vi "test Call Mock Transceiver With Errors.vi"(8 "error in (no error)":errorcluster, 11 "TestCase in":refnum<class "Transceiver Test Cases.lvclass">) -> (0 "error out":errorcluster, 3 "TestCase out":refnum<class "Transceiver Test Cases.lvclass">)   [LabVIEW 2017, in "Transceiver Test Cases.lvclass"]
uses:
  Transceiver Test Cases.lvclass
  Configuration/Public/Controls/DSF Engine Transfer Group Configuration.ctl
  Configuration/Public/Controls/DSF Direction.ctl
  Configuration/Public/Controls/DSF Timing Info.ctl
  Configuration/Public/Controls/DSF Engine Transfer Configuration.ctl
  Configuration/Public/Controls/DSF Byte Order.ctl
  Configuration/Public/Controls/DSF Engine Channel Configuration.ctl
  Configuration/Public/Controls/DSF Data Type.ctl
  Configuration/Public/Controls/DSF Settings Info.ctl
  DSF Core.lvlib
  <vilib>/addons/_JKI Toolkits/VI Tester/TestCase.llb/TestCase.lvclass
  C:/Program Files (x86)/National Instruments/LabVIEW 2017/vi.lib/addons/_JKI Toolkits/VI Tester/TestCase.llb/TestCase.lvclass
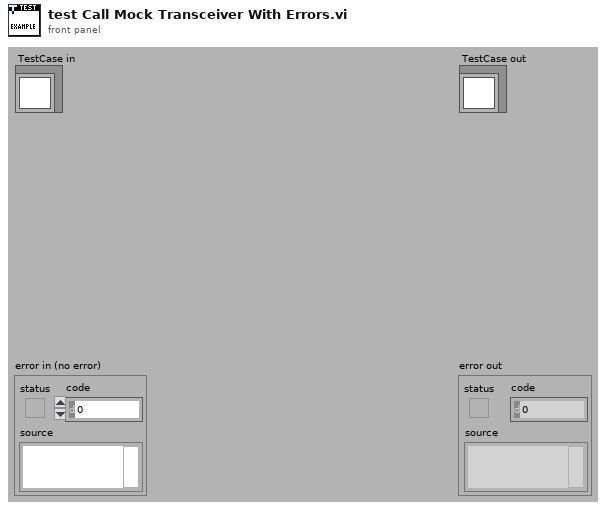
[diagram p1: front panel]
types:
  T1 = typedef "DSF Core.lvlib/DSF Engine Transfer Group Configuration.ctl" = cluster{"name":string, "direction":T2, "cycle timing":T3, "Transfers":T4[], "settings":T8}
  T2 = typedef "DSF Core.lvlib/DSF Direction.ctl" = enum8{"Tx", "Rx"}
  T3 = typedef "DSF Core.lvlib/DSF Timing Info.ctl" = cluster{"priority":u64, "decimation":u64, "offset":u64}
  T4 = typedef "DSF Core.lvlib/DSF Engine Transfer Configuration.ctl" = cluster{"name":string, "byte order":T5, "channel configurations":T6[], "settings":T8}
  T5 = typedef "DSF Core.lvlib/DSF Byte Order.ctl" = enum8{"big-endian", "little-endian"}
  T6 = typedef "DSF Core.lvlib/DSF Engine Channel Configuration.ctl" = cluster{"engine offset":u64, "name":string, "data type":T7, "count":u64, "buffer offset":u64}
  T7 = typedef "DSF Core.lvlib/DSF Data Type.ctl" = enum8{"Bool", "SGL", "DBL", "I8", "I16", "I32", "I64", "U8", "U16", "U32", "U64"}
  T8 = typedef "DSF Core.lvlib/DSF Settings Info.ctl" = cluster{"key":string, "value":string}[]
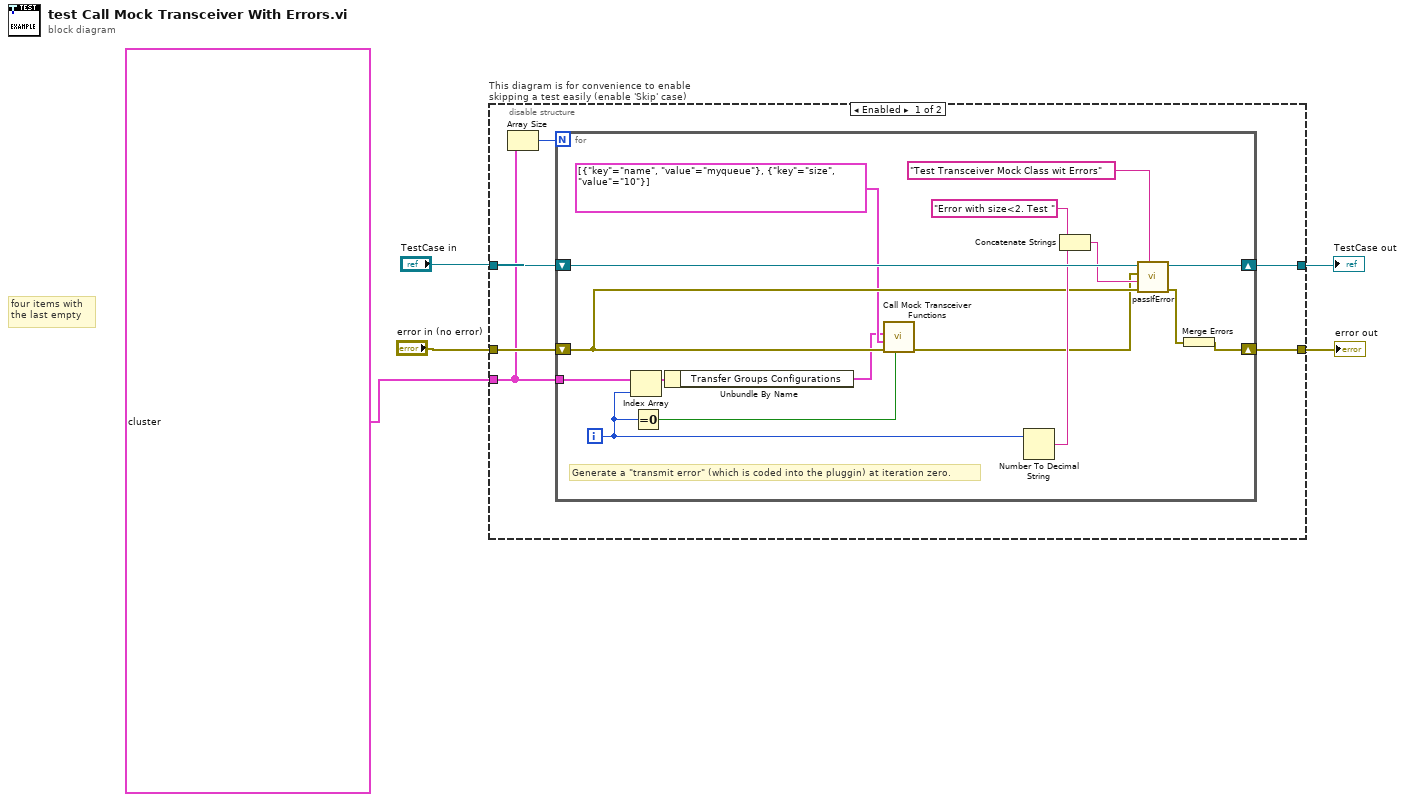
[diagram p0: block diagram]
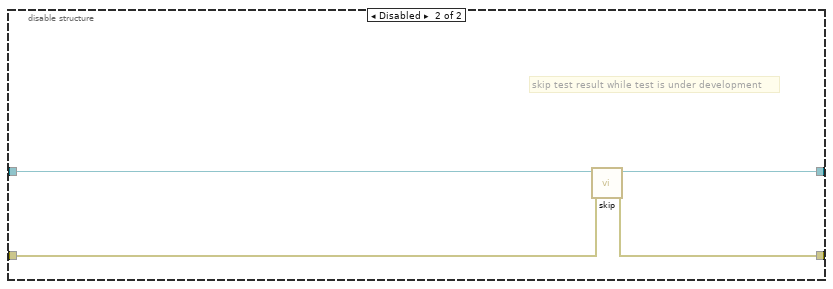
[diagram p2: hidden frame]
diagram:
  # "four items with \nthe last empty"
  n1 = disable-structure "This diagram is for convenience to enable skipping a test easily (enable 'Skip' case)" shown="Enabled" {
    disable-tunnel: "TestCase in" -> [w11 w31]
    disable-tunnel: [w9 w29] -> w4
    disable-tunnel: [w10 w30] -> w3
    disable-tunnel: "error in (no error)" -> [w8 w28]
    disable-tunnel: cluster{"Transfer Groups Configurations":T1[]}[] [{"Transfer Groups Configurations"=[{"name"="", "direction"=enum."Tx", "cycle timing"={"priority"=0, "decimation"=1, "offset"=0}, "Transfers"=[], "settings"=[]}, {"name"="", "direction"=enum."Rx", "cycle timing"={"priority"=0, "decimation"=1, "offset"=0}, "Transfers"=[], "settings"=[]}]}, {"Transfer Groups Configurations"=[{"name"="", "direction"=enum."Tx", "cycle timing"={"priority"=0, "decimation"=1, "offset"=0}, "Transfers"=[], "settings"=[]}]}, {"Transfer Groups Configurations"=[{"name"="", "direction"=enum."Rx", "cycle timing"={"priority"=0, "decimation"=1, "offset"=0}, "Transfers"=[], "settings"=[]}]}, {"Transfer Groups Configurations"=[]}] -> [w7 _]
    frame Enabled {
      n2 = Array Size(array=w7) -> (size(s)=w6:i32)
      n3 = for {
        N: w6 -> [_]
        shift-right: [w23] -> w9
        shift-left: w11 -> [w25]
        shift-right: [w24] -> w10
        shift-left: w8 -> [w19]
        tunnel: w7 -> [w16]
        i -> [w12]
        # "Generate a \"transmit error\" (which is coded into the pluggin) at iteration zero."
        n4 = Index Array(array=w16, index=w12) -> (element=w14:cluster{"Transfer Groups Configurations":T1[]})
        n5 = Equal To 0?(x=w12) -> (x = 0?=w13:bool)
        n6 = Unbundle By Name(w14) -> ("Transfer Groups Configurations"=w15:T1[])
        n7 = call "Call Mock Transceiver Functions.vi"("Fail to transmit?"=w13, "error in"=w19, "transceiver settings"=T8 [{"key"="name", "value"="myqueue"}, {"key"="size", "value"="10"}], "Transfer Groups Configurations"=w15) -> ("error out"=w18:errorcluster)  [unwired: 6 in, 1 out]
        n8 = Number To Decimal String(number=w12) -> (decimal integer string=w21:string)  [unwired: 1 in]
        n9 = Concatenate Strings("Error with size<2. Test " ("custom report message (\"\")"), w21) -> (w20:string)
        n10 = call-dynamic "passIfError.vi"("custom report message (\"\")"="Test Transceiver Mock Class wit Errors" ("custom report message (\"\")"), "error in (no error)"=w19, "task (\"\")"=w20, "error"=w18, "TestCase in"=w25) -> ("error out"=w27:errorcluster, "TestCase out"=w23:refnum<class "Transceiver Test Cases.lvclass">)  [unwired: 5 in]
        n11 = Merge Errors(w27) -> (w24:errorcluster)
      }
    }
    frame Disabled {
      # "skip test result while test is under development"
      n12 = call <vilib>:"skip.vi"("error in (no error)"=w28, "TestCase in"=w31) -> ("error out"=w30:errorcluster, "TestCase out"=w29:refnum<class "Transceiver Test Cases.lvclass">)  [unwired: 8 in]
    }
  }
  "error out" <- w3
  "TestCase out" <- w4
